vi "Zero_Offset_Channel_Names.vi"(7 "Calib Filename":path) -> (0 "Channel names":string[](array[string]), 1 "Voltage Index":i32, 2 "Time Index":i32, 3 "Zero Filename":path)   [LabVIEW 2022 SP3]
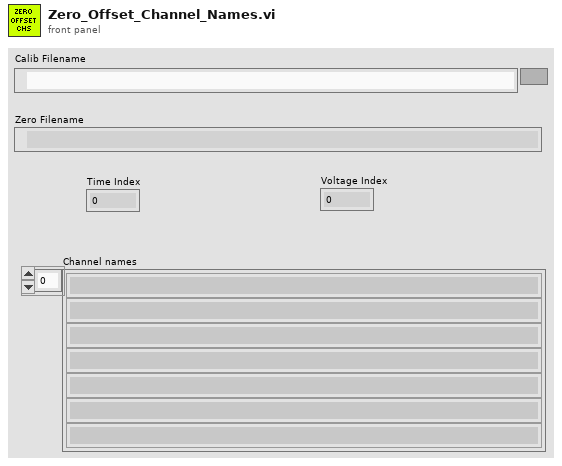
[diagram p1: front panel]
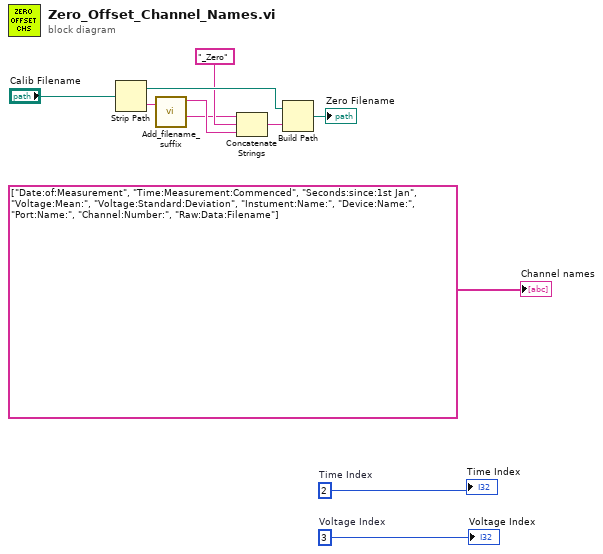
[diagram p0: block diagram]
diagram:
  w1 = 3  # Voltage Index
  w2 = 2  # Time Index
  n1 = Strip Path(path="Calib Filename") -> (stripped path=w9:path, name=w5:string)
  n2 = call "Add_filename_suffix.vi"("Filename"=w5) -> ("Original Suffix"=w8:string, "Base name"=w6:string)  [unwired: 1 in, 2 out]
  n3 = Concatenate Strings(w6, "_Zero" ("string"), w8) -> (w10:string)
  n4 = Build Path(base path=w9, name or relative path=w10) -> (appended path=→"Zero Filename":path)
  "Channel names" <- string[] ["Date:of:Measurement", "Time:Measurement:Commenced", "Seconds:since:1st Jan", "Voltage:Mean:", "Voltage:Standard:Deviation", "Instument:Name:", "Device:Name:", "Port:Name:", "Channel:Number:", "Raw:Data:Filename"] ("Channel names")
  "Time Index" <- w2
  "Voltage Index" <- w1
